vi "scale_to_max.vi"(8 "error in (no error)":errorcluster, 10 "max length (pixels)":i32=200, 11 "Image in":refnum<class "Image.lvclass">) -> (0 "error out":errorcluster, 3 "Image out":refnum<class "Image.lvclass">)   [LabVIEW 2010, in "Image.lvclass"]
uses:
  Image.lvclass
  ErrorController/ErrorController/class_data.vi
  ErrorController/ErrorController/ErrorController.lvclass
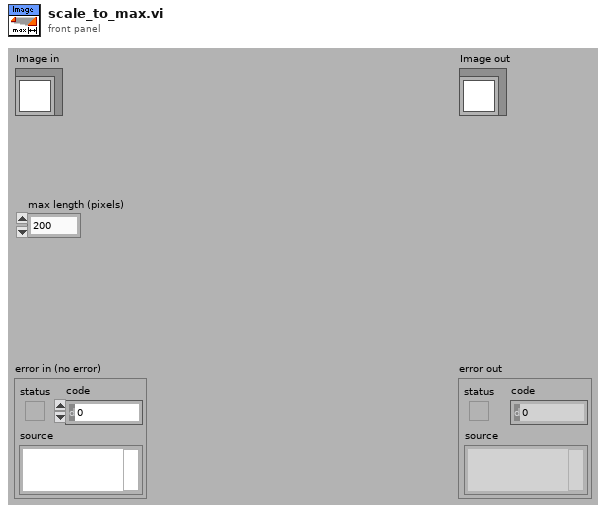
[diagram p1: front panel]
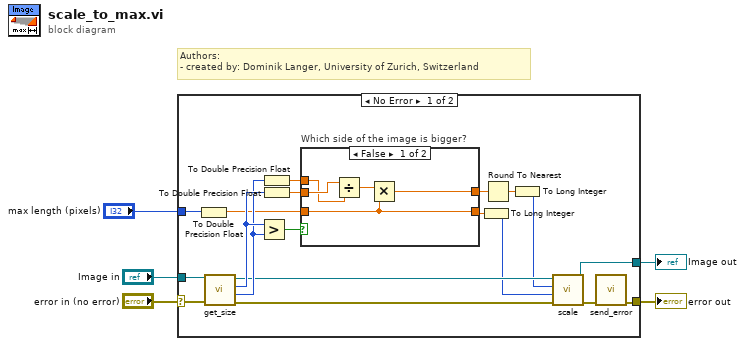
[diagram p0: block diagram]
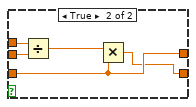
[diagram p2: hidden frame]
diagram:
  # "Authors: \n- created by: Dominik Langer, University of Zurich, Switzerland"
  n1 = case shown="No Error" "error in (no error)" {
    selector: "error in (no error)" -> [w23 w36]
    tunnel: [w6 w36] -> w4
    tunnel: [w15 w35] -> w2
    tunnel: "Image in" -> [w24 w35]
    tunnel: "max length (pixels)" -> [w14 _]
    frame No Error {
      n2 = To Double Precision Float(number=w14) -> (double precision float=w13:dbl)
      n3 = call-dynamic "get_size.vi"("error in (no error)"=w23, "Image in"=w24) -> ("error out"=w17:errorcluster, "y resolution"=w19:i32, "x resolution"=w20:i32, "Image out"=w16:refnum<class "Image.lvclass">)  [unwired: 6 out]
      n4 = Greater?(x=w20, y=w19) -> (0:w22:bool)
      n5 = To Double Precision Float(number=w19) -> (double precision float=w21:dbl)
      n6 = To Double Precision Float(number=w20) -> (double precision float=w18:dbl)
      n7 = case "Which side of the image is bigger?" shown="False" w22 {
        tunnel: w21 -> [w28 w34]
        tunnel: w13 -> [w27 w31]
        tunnel: [w27 w30] -> w12
        tunnel: w18 -> [w29 w33]
        tunnel: [w25 w31] -> w10
        frame False {
          n8 = Divide(x=w29, y=w28) -> (x/y=w26:dbl)
          n9 = Multiply(x=w26, y=w27) -> (x*y=w25:dbl)
        }
        frame True {
          n10 = Divide(x=w34, y=w33) -> (x/y=w32:dbl)
          n11 = Multiply(x=w32, y=w31) -> (x*y=w30:dbl)
        }
      }
      n12 = To Long Integer(number=w12) -> (32bit integer=w11:i32)
      n13 = Round To Nearest(number=w10) -> (nearest integer value=w9:dbl)
      n14 = To Long Integer(number=w9) -> (32bit integer=w8:i32)
      n15 = call-dynamic "scale.vi"("error in (no error)"=w17, "y"=w11, "x"=w8, "Image in"=w16) -> ("error out"=w7:errorcluster, "Image out"=w15:refnum<class "Image.lvclass">)  [unwired: 6 out]
      n16 = call "send_error.vi"("error in (no error)"=w7) -> ("error out"=w6:errorcluster)  [unwired: 10 in]
    }
    frame Error {
    }
  }
  "error out" <- w4
  "Image out" <- w2
